vi "Config Wideband CDMA.vi"(0 "VISA Resource Name":refnum<visa-resource-name>, 1 "Long Code (1)":i32=1, 2 "ARB Reference (F:INT)":bool, 3 "Reference Freq (10.0)":dbl=10.0 format="%.8f", 5 "PERCH1 (F:OFF)":bool, 7 "DTCH Channels (1)":i32=1, 9 "DTCH Symbols (2:FMTD OFFSET)":T1(ring)=enum."FORMATTED ALIGNED", 11 "error in (no error)":errorcluster {"code" format="%.0x"}) -> (4 "VISA Resource Name Out":refnum<visa-resource-name>, 15 "error out":errorcluster {"code" format="%.0x"})   [LabVIEW 2012, in "Agilent ESG Series.lvlib"]
doc: "This VI is used to configure the Wideband CDMA option.\n\nThis VI is valid only on instruments with the UND and UN5 options."
uses:
  <instrlib>/Agilent ESG Series/Agilent ESG Series.lvlib
panel:
  # "ON"
  # "OFF"
  # "EXT"
  # "INT"
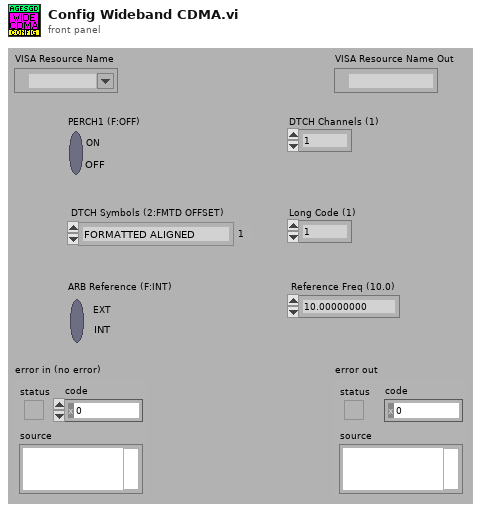
[diagram p1: front panel]
types:
  T1 = enum16{"RANDOM", "FORMATTED ALIGNED", "FORMATTED OFFSET"}
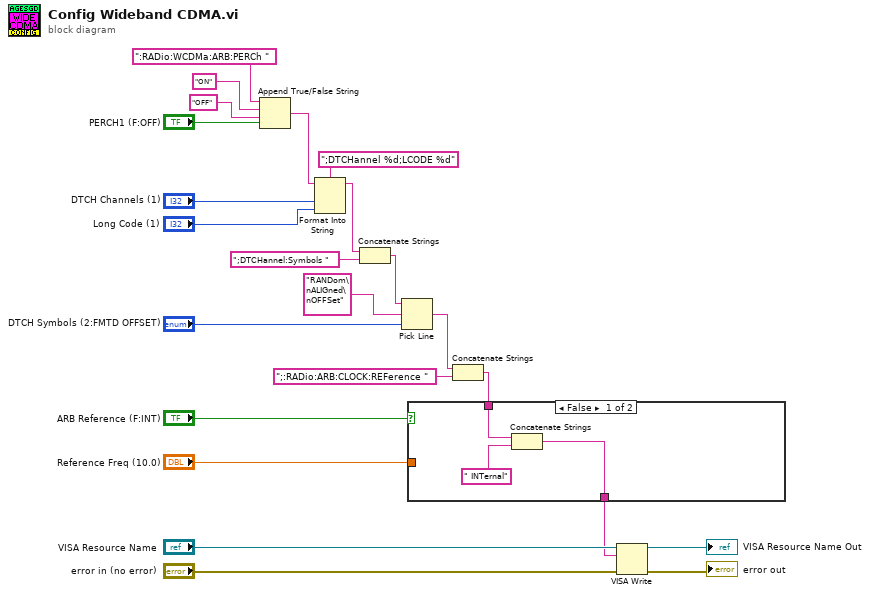
[diagram p0: block diagram]
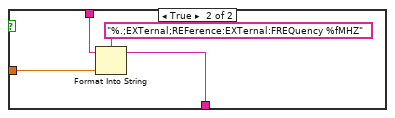
[diagram p2: hidden frame]
diagram:
  n1 = Append True/False String(1:"PERCH1 (F:OFF)", 2:"OFF", 3:"ON", 4:":RADio:WCDMa:ARB:PERCh " ("string (\"\")")) -> (0:w2:string)
  n2 = Format Into String(format string=";DTCHannel %d;LCODE %d", initial string=w2, "DTCH Channels (1)", "Long Code (1)") -> (resulting string=w3:string)  [unwired: 1 in, 1 out]
  n3 = Concatenate Strings(w3, ";DTCHannel:Symbols " ("string (\"\")")) -> (w5:string)
  n4 = Pick Line(string ("")=w5, multi-line string="RANDom\nALIGned\nOFFSet", line index="DTCH Symbols (2:FMTD OFFSET)") -> (output string=w1:string)
  n5 = Concatenate Strings(w1, ";:RADio:ARB:CLOCK:REFerence " ("string (\"\")")) -> (w17:string)
  n6 = case shown="False" "ARB Reference (F:INT)" {
    tunnel: w17 -> [w26 w30]
    tunnel: [w24 w27] -> w14
    tunnel: "Reference Freq (10.0)" -> [_ w28]
    frame False {
      n7 = Concatenate Strings(w26, " INTernal") -> (w24:string)
    }
    frame True {
      n8 = Format Into String(format string="%.;EXTernal;REFerence:EXTernal:FREQuency %fMHZ", initial string=w30, w28) -> (resulting string=w27:string)  [unwired: 1 in, 1 out]
    }
  }
  n9 = VISA Write(VISA resource name="VISA Resource Name", write buffer=w14, error in (no error)="error in (no error)") -> (VISA resource name out=→"VISA Resource Name Out":refnum<visa-resource-name>, error out=→"error out":errorcluster)  [unwired: 1 out]
